vi "Main.vi"() -> ()   [LabVIEW 2015]
doc: "This template is for the Queued Message Handler design pattern.\n\nThe Event Handling Loop generates messages based on user interface actions.\n\nThe Message Handling Loop processes messages generated by the Event Handling Loop, or by other messages. The messages are string values, so new messages can be added easily to the Message Cases case structure in the Message Handling Loop. Each message cluster can also provide an optional value for Message Data, which is a variant that can be converted to whatever message-specific data is required."
uses:
  controls/UI Data.ctl
  support/Boiler System Globals.vi
  support/Message Queue/Message Queue.lvlib
  support/User Event - Stop/User Event - Stop.lvlib
panel:
  out "Display <Replace Me>":string
  in  "Do Something Else <Replace Me>":bool
  in  "Do Something <Replace Me>":bool
  in  "Stop Button":bool
  # "These controls have associated \"Value Changed\" events configured in the Event Structure on the diagram.\n\nReplace them (and reconfigure the Event Structure) with the controls you need for your application."
  # "This template is for the Queued Message Handler design pattern.\n\nSee the block diagram for more information on how to use this template."
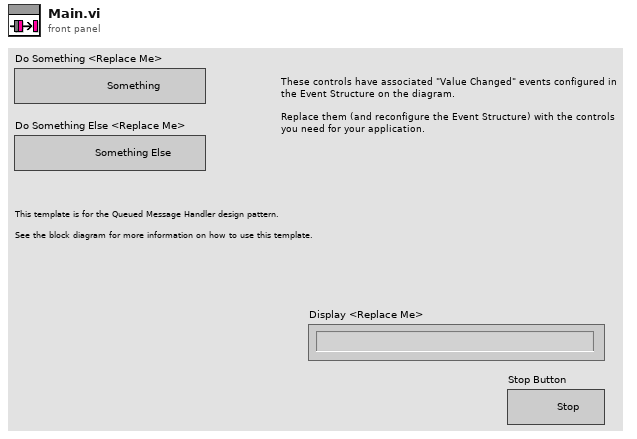
[diagram p1: front panel]
types:
  T1 = typedef "UI Data.ctl" = cluster{"Boolean <Replace Me>":bool, "String <Replace Me>":string, "Numeric <Replace Me>":dbl, "Do Something Ref":refnum<vi>, "Do Something Else Ref":refnum<vi>, "Data Display Ref":refnum<vi>, "Stop Button Ref":refnum<vi>}
  T2 = typedef "Message Queue.lvlib/All Message Queues.ctl" = cluster{"MHL":refnum<queue>, "Boiler Controler":refnum<queue>}
  T3 = enum32{"invalid app kind", "Development System", "Run Time System", "Student Edition", "Embedded LabVIEW", "Evaluation", "Custom"}
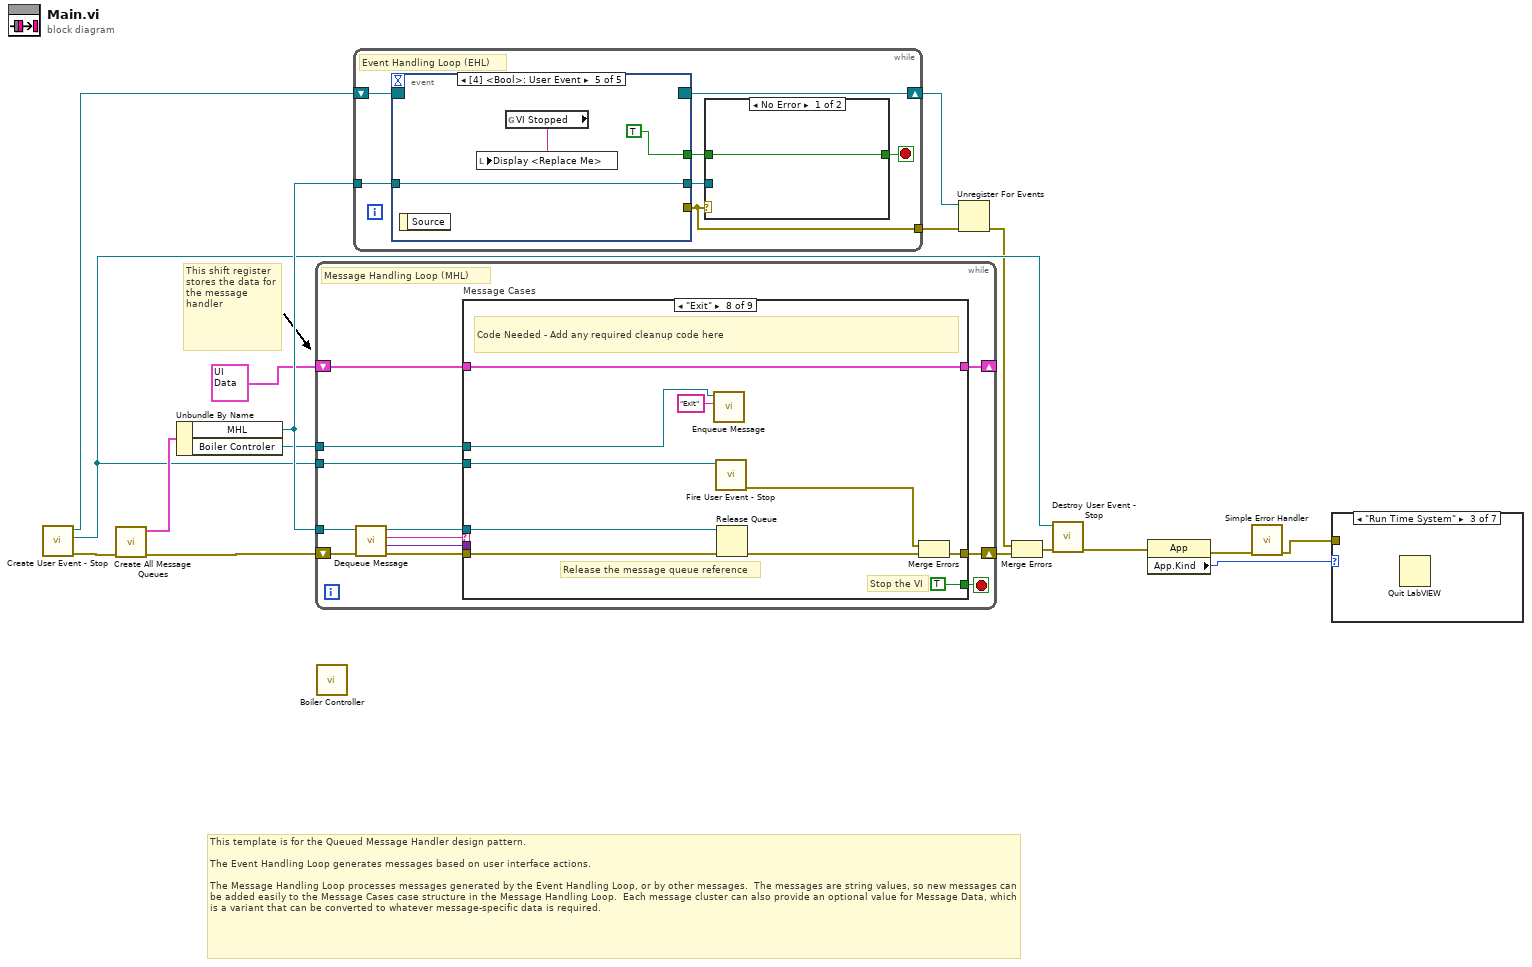
[diagram p0: block diagram]
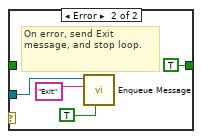
[diagram p8: hidden frame]
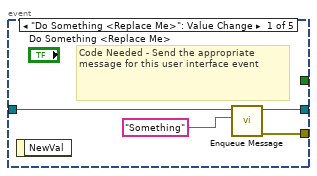
[diagram p9: hidden frame]
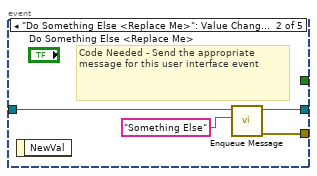
[diagram p10: hidden frame]
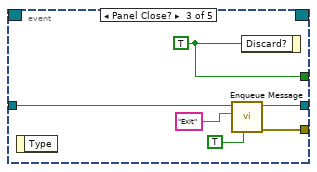
[diagram p11: hidden frame]
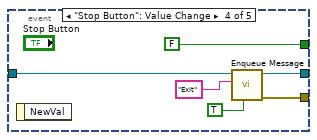
[diagram p12: hidden frame]
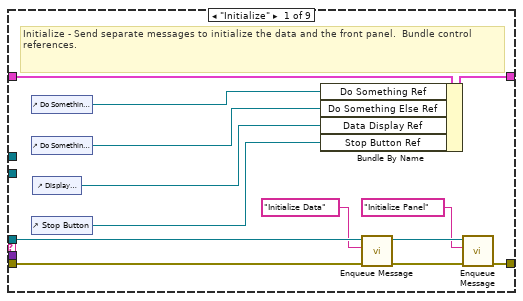
[diagram p13: hidden frame]
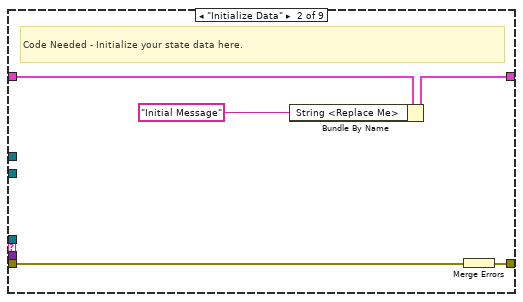
[diagram p14: hidden frame]
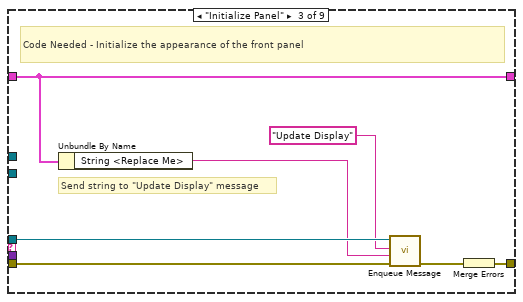
[diagram p15: hidden frame]
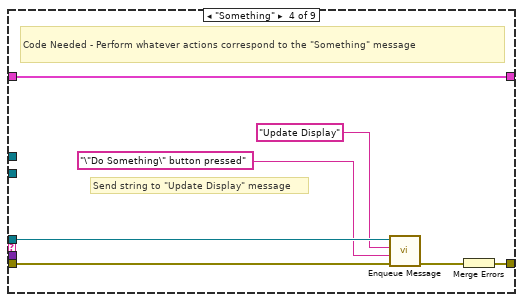
[diagram p16: hidden frame]
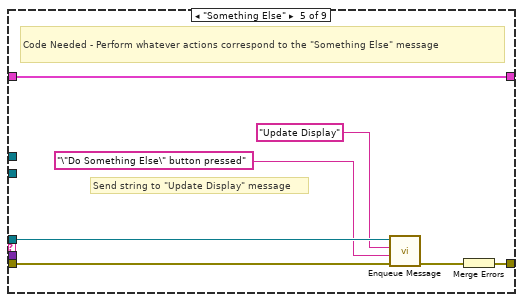
[diagram p17: hidden frame]
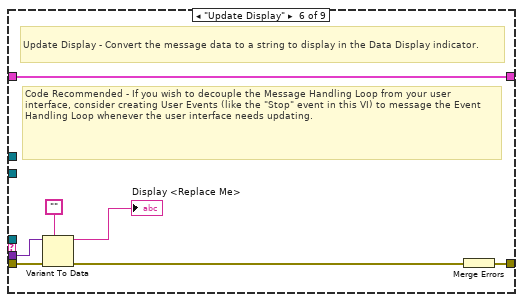
[diagram p18: hidden frame]
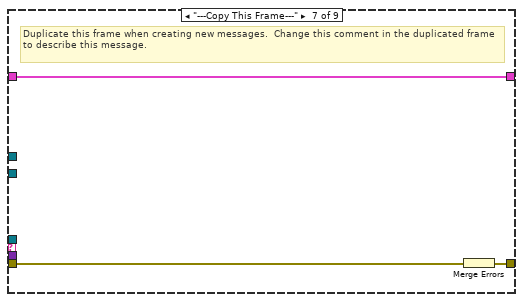
[diagram p19: hidden frame]
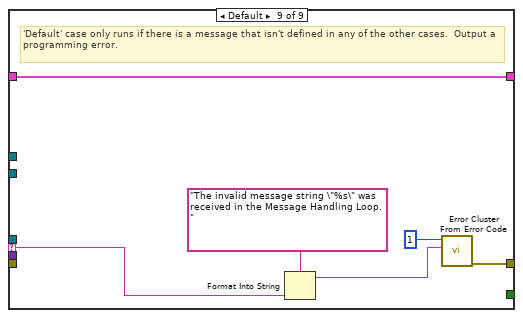
[diagram p20: hidden frame]
diagram:
  # "This template is for the Queued Message Handler design pattern.\n\nThe Event Handling Loop generates messages based on user interface actions.\n\nThe Message Handling Loop processes messages generated by the Event Handling Loop, or by other messages.  The messages are string values, so new messages can be added easily to the Message Cases case structure in the Message Handling Loop.  Each message cluster can also provide an optional value for Message Data, which is a variant that can be converted to whatever message-specific data is required."
  # "This shift register\nstores the data for the message handler"
  n1 = call "Create User Event - Stop.vi"() -> ("error out"=w13:errorcluster, "User bool - Stop"=w11:refnum<user-event>, "Event Registration Refnum"=w6:refnum<event-registration>)  [unwired: 9 in]
  n2 = call "Create All Message Queues.vi"("error in (no error)"=w13) -> ("error out"=w17:errorcluster, "Message Queues out"=w16:T2)  [unwired: 9 in]
  n3 = Unbundle By Name(w16) -> ("MHL"=w14:refnum<queue>, "Boiler Controler"=w5:refnum<queue>)
  n4 = while {
    tunnel: w14 -> [w19]
    shift-right: [w28] -> _
    shift-left: T1 {"Boolean <Replace Me>"=TRUE, "String <Replace Me>"="", "Numeric <Replace Me>"=0.0, "Do Something Ref"=refnum, "Do Something Else Ref"=refnum, "Data Display Ref"=refnum, "Stop Button Ref"=refnum} ("Data Cluster") -> [w29]
    tunnel: w11 -> [w25]
    shift-right: [w26] -> w15
    shift-left: w17 -> [w24]
    tunnel: w5 -> [w18]
    stop <- w27 stop-if-true
    # "Message Handling Loop (MHL)"
    n5 = call "Dequeue Message.vi"("error in (no error)"=w24, "Message Queue"=w19) -> ("error out"=w23:errorcluster, "Message Data"=w21:variant, "Message"=w22:string, "dup Message Queue"=w20:refnum<queue>)  [unwired: 6 in]
    n6 = case "Message Cases" shown="\"Exit\"" w22 {
      selector: w22 -> [_ _ _ _ _ _ _ _ w92]
      tunnel: w20 -> [w38 _ w51 w57 w64 _ _ w88 _]
      tunnel: w23 -> [w41 w47 w52 w59 w66 w73 w78 w83 _]
      tunnel: [w42 w43 w53 w60 w67 w74 w76 w84 w90] -> w26
      tunnel: w29 -> [w35 w46 w54 w61 w68 w75 w77 w87 w94]
      tunnel: [w34 w45 w54 w61 w68 w75 w77 w87 w94] -> w28
      tunnel: [_ _ _ _ _ _ _ TRUE _] -> w27
      tunnel: w21 -> [_ _ _ _ _ w72 _ _ _]
      tunnel: w25 -> [_ _ _ _ _ _ _ w82 _]
      tunnel: w18 -> [_ _ _ _ _ _ _ w79 _]
      frame "Initialize" {
        # "Initialize - Send separate messages to initialize the data and the front panel.  Bundle control references."
        n7 = control-ref of="Do Something <Replace Me>"() -> (w33:refnum<vi>)
        n8 = control-ref of="Do Something Else <Replace Me>"() -> (w32:refnum<vi>)
        n9 = control-ref of="Stop Button"() -> (w30:refnum<vi>)
        n10 = control-ref of="Display <Replace Me>"() -> (w31:refnum<vi>)
        n11 = Bundle By Name(cluster=w35, "Do Something Ref"=w33, "Do Something Else Ref"=w32, "Data Display Ref"=w31, "Stop Button Ref"=w30) -> (w34:T1)
        n12 = call "Enqueue Message.vi"("error in (no error)"=w41, "Message"="Initialize Data", "Message Queue"=w38) -> ("error out"=w40:errorcluster, "dup Message Queue"=w39:refnum<queue>)  [unwired: 7 in]
        n13 = call "Enqueue Message.vi"("error in (no error)"=w40, "Message"="Initialize Panel", "Message Queue"=w39) -> ("error out"=w42:errorcluster)  [unwired: 7 in, 1 out]
      }
      frame "Initialize Data" {
        # "Code Needed - Initialize your state data here."
        n14 = Bundle By Name(cluster=w46, "String <Replace Me>"="Initial Message" ("Initial Message")) -> (w45:T1)
        n15 = Merge Errors(w47) -> (w43:errorcluster)
      }
      frame "Initialize Panel" {
        # "Send string to \"Update Display\" message"
        # "Code Needed - Initialize the appearance of the front panel"
        n16 = Unbundle By Name(w54) -> ("String <Replace Me>"=w48:string)
        n17 = call "Enqueue Message.vi"("error in (no error)"=w52, "Message Data"=w48, "Message"="Update Display", "Message Queue"=w51) -> ("error out"=w50:errorcluster)  [unwired: 6 in, 1 out]
        n18 = Merge Errors(w50) -> (w53:errorcluster)
      }
      frame "Something" {
        # "Send string to \"Update Display\" message"
        # "Code Needed - Perform whatever actions correspond to the \"Something\" message"
        n19 = call "Enqueue Message.vi"("error in (no error)"=w59, "Message Data"="\"Do Something\" button pressed" ("\"Do Something\" button pressed"), "Message"="Update Display", "Message Queue"=w57) -> ("error out"=w58:errorcluster)  [unwired: 6 in, 1 out]
        n20 = Merge Errors(w58) -> (w60:errorcluster)
      }
      frame "Something Else" {
        # "Send string to \"Update Display\" message"
        # "Code Needed - Perform whatever actions correspond to the \"Something Else\" message"
        n21 = call "Enqueue Message.vi"("error in (no error)"=w66, "Message Data"="\"Do Something Else\" button pressed" ("\"Do Something Else\" button pressed"), "Message"="Update Display", "Message Queue"=w64) -> ("error out"=w65:errorcluster)  [unwired: 6 in, 1 out]
        n22 = Merge Errors(w65) -> (w67:errorcluster)
      }
      frame "Update Display" {
        # "Code Recommended - If you wish to decouple the Message Handling Loop from your user interface, consider creating User Events (like the \"Stop\" event in this VI) to message the Event Handling Loop whenever the user interface needs updating."
        # "Update Display - Convert the message data to a string to display in the Data Display indicator."
        n23 = Variant To Data(error in=w73, type="", Variant=w72) -> (data=→"Display <Replace Me>":string, error out=w70:errorcluster)
        n24 = Merge Errors(w70) -> (w74:errorcluster)
      }
      frame "---Copy This Frame---" {
        # "Duplicate this frame when creating new messages.  Change this comment in the duplicated frame to describe this message."
        n25 = Merge Errors(w78) -> (w76:errorcluster)
      }
      frame "Exit" {
        # "Stop the VI"
        # "Release the message queue reference"
        # "Code Needed - Add any required cleanup code here"
        n26 = call "Enqueue Message.vi"("Message"="Exit", "Message Queue"=w79) -> ()  [unwired: 8 in, 2 out]
        n27 = call "Fire User Event - Stop.vi"("User Event - Stop"=w82) -> ("error out"=w81:errorcluster)  [unwired: 10 in]
        n28 = Release Queue(queue=w88, error in (no error)=w83) -> (error out=w85:errorcluster)  [unwired: 1 in, 2 out]
        n29 = Merge Errors(w81, w85) -> (w84:errorcluster)
      }
      frame Default {
        # "'Default' case only runs if there is a message that isn't defined in any of the other cases.  Output a programming error."
        n30 = Format Into String(format string="The invalid message string \"%s\" was received in the Message Handling Loop." ("Unknown Message Error Text"), w92) -> (resulting string=w89:string)  [unwired: 2 in, 1 out]
        n31 = call <vilib>:"Error Cluster From Error Code.vi"("error message (\"\")"=w89, "error code (0)"=1) -> ("error out"=w90:errorcluster)  [unwired: 7 in]
      }
    }
  }
  n32 = call "Boiler Controller.vi"() -> ()  [unwired: 11 in, 1 out]
  n33 = while {
    tunnel: w14 -> [w101]
    tunnel: [w97] -> w9
    shift-right: [w96] -> w8
    shift-left: w6 -> [w95]
    stop <- w99 stop-if-true
    # "Event Handling Loop (EHL)"
    n34 = event shown="[4] <Bool>: User Event" {
      selector: w95 -> [_ _ _ _ _]
      dyn-events: [_ _ _ _ _] -> w96
      timeout: _ -> [_ _ _ _ _]
      tunnel: [_ _ w120 FALSE ("Discard?") TRUE] -> w100
      tunnel: w101 -> [w110 w114 w119 w126 w129]
      tunnel: [w109 w112 w118 w125 _] -> w97
      tunnel: [w108 w113 w117 w123 w129] -> w98
      event "Do Something <Replace Me>": Value Change {
        # "Code Needed - Send the appropriate message for this user interface event"
        n35 = event-data() -> ()  [unwired: 1 in, 1 out]
        n36 = call "Enqueue Message.vi"("Message"="Something", "Message Queue"=w110) -> ("error out"=w109:errorcluster, "dup Message Queue"=w108:refnum<queue>)  [unwired: 8 in]
      }
      event "Do Something Else <Replace Me>": Value Change {
        # "Code Needed - Send the appropriate message for this user interface event"
        n37 = event-data() -> ()  [unwired: 1 in, 1 out]
        n38 = call "Enqueue Message.vi"("Message"="Something Else", "Message Queue"=w114) -> ("error out"=w112:errorcluster, "dup Message Queue"=w113:refnum<queue>)  [unwired: 8 in]
      }
      event Panel Close? {
        w120 = TRUE ("Discard?")
        n39 = event-data() -> ()  [unwired: 1 in, 1 out]
        n40 = call "Enqueue Message.vi"("Priority Message? (F)"=TRUE, "Message"="Exit", "Message Queue"=w119) -> ("error out"=w118:errorcluster, "dup Message Queue"=w117:refnum<queue>)  [unwired: 7 in]
        n41 = event-data("Discard?"=w120) -> ()  [unwired: 1 in, 1 out]
      }
      event "Stop Button": Value Change {
        n42 = event-data() -> ()  [unwired: 1 in, 1 out]
        n43 = call "Enqueue Message.vi"("Priority Message? (F)"=TRUE, "Message"="Exit", "Message Queue"=w126) -> ("error out"=w125:errorcluster, "dup Message Queue"=w123:refnum<queue>)  [unwired: 7 in]
      }
      event User Event {
        n44 = event-data() -> ()  [unwired: 1 in, 1 out]
        n45 = global read "Boiler System Globals.vi" "VI Stopped"() -> (w128:string)
        n46 = local write "Display <Replace Me>"(w128) -> ()
      }
    }
    n47 = case shown="No Error" w97 {
      tunnel: [w102 TRUE ("Discard?")] -> w99
      tunnel: w100 -> [w102 _]
      tunnel: w98 -> [_ w105]
      frame No Error {
      }
      frame Error {
        # "On error, send Exit message, and stop loop."
        n48 = call "Enqueue Message.vi"("Priority Message? (F)"=TRUE, "Message"="Exit", "Message Queue"=w105) -> ()  [unwired: 7 in, 2 out]
      }
    }
  }
  n49 = Unregister For Events(event registration refnum=w8, error in=w9) -> (error out=w10:errorcluster)
  n50 = Merge Errors(w10, w15) -> (w12:errorcluster)
  n51 = call "Destroy User Event - Stop.vi"("error in (no error)"=w12, "User Event - Stop"=w11) -> ("error out"=w4:errorcluster)  [unwired: 9 in]
  n52 = property class="App"(error in=w4) -> (error out=w3:errorcluster, "App.Kind"=w2:T3)  [unwired: 1 in, 1 out]
  n53 = call <vilib>:"Simple Error Handler.vi"("error in (no error)"=w3) -> ("error out"=w1:errorcluster)  [unwired: 4 in, 4 out]
  n54 = case shown="\"Run Time System\"" w2 {
    tunnel: w1 -> [_ _ _ _ _ _ _]
    frame "invalid app kind", Default {
    }
    frame "Development System" {
    }
    frame "Run Time System" {
      n55 = Quit LabVIEW() -> ()  [unwired: 1 in]
    }
    frame "Student Edition" {
    }
    frame "Embedded LabVIEW" {
    }
    frame "Evaluation" {
    }
    frame "Custom" {
    }
  }
